vi "Monitor_Temp.vi"(2 "Debug Mode":bool, 3 "Elapsed Time (s)":dbl, 4 "State":enum16{"Edit", "Start", "Run", "End", "Idle"}(ring), 5 "Argument List In":string[](array[string])) -> (0 "Status Out":string, 1 "Argument List Out":string[](array[string]))   [LabVIEW 2011]
panel:
  in  "Cancel":bool
  in  "OK":bool
  out "Temperature":dbl
  out "Read Cycle":dbl
  out "Timer":dbl
  out "Previous Time":dbl
  in  "Target (C)":dbl
  # "Wait for this target \nto be reached."
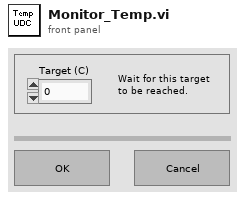
[diagram p1: front panel]
types:
  T1 = enum16{"Discrete", "Continuous", "Instantaneous"}
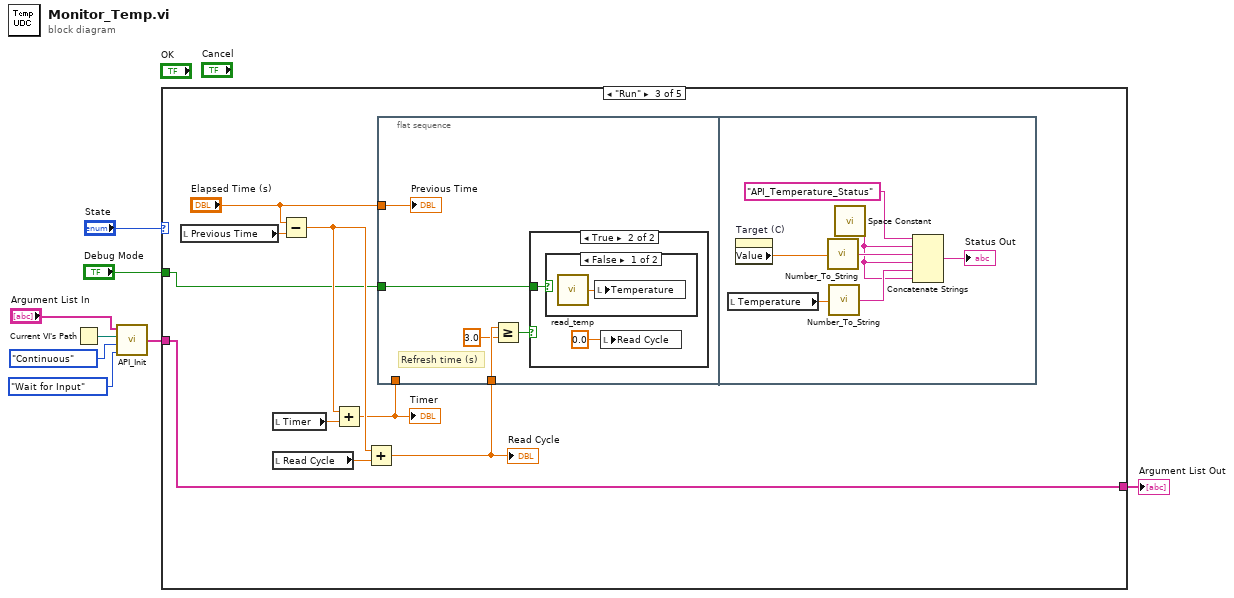
[diagram p0: block diagram]
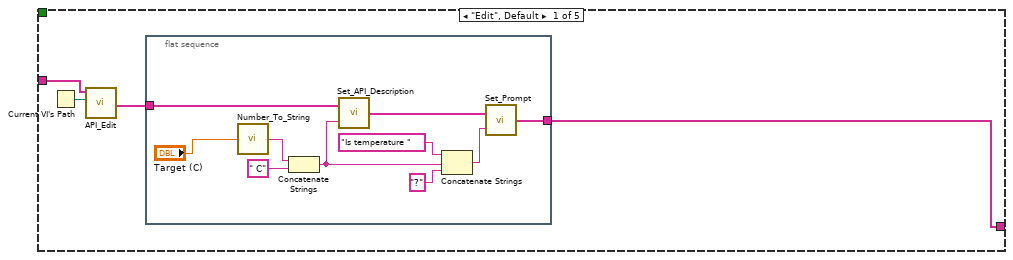
[diagram p2: hidden frame]
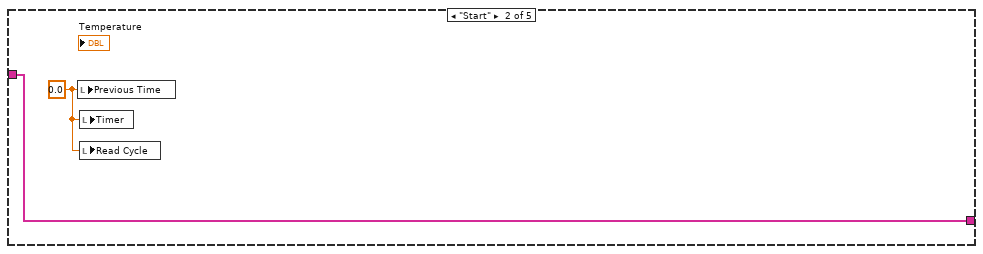
[diagram p3: hidden frame]
diagram:
  n1 = Current VI's Path() -> (path=w5:path)
  n2 = call "API_Init.vi"("API Option"=enum16{"None", "Blocking", "Wait for Input"}."Wait for Input", "API Mode"=T1."Continuous", "VI Path"=w5, "Argument List In"="Argument List In") -> ("Argument List Out"=w2:string[])
  n3 = case shown="\"Run\"" "State" {
    tunnel: [w9 w24 w33 w49 w50] -> w7
    tunnel: w2 -> [w11 w24 w33 w49 w50]
    tunnel: "Debug Mode" -> [_ _ w25 _ _]
    frame "Edit", Default {
      n4 = Current VI's Path() -> (path=w12:path)
      n5 = call "API_Edit.vi"("VI Path"=w12, "Argument List In"=w11) -> ("Argument List Out"=w10:string[])  [unwired: 2 in]
      n6 = flat-sequence {
        tunnel: w10 -> [w16]
        tunnel: [w14] -> w9
        frame #0 {
          n7 = call "Number_To_String.vi"("Number"="Target (C)") -> ("String"=w15:string)
          n8 = Concatenate Strings(w15, " C" ("string")) -> (w20:string)
          n9 = call "Set_API_Description.vi"("Description"=w20, "Argument List In"=w16) -> ("Argument List Out"=w21:string[])
          n10 = Concatenate Strings("Is temperature " ("Prompt"), w20, "?" ("string")) -> (w17:string)
          n11 = call "Set_Prompt.vi"("Prompt"=w17, "Argument List In"=w21) -> ("Argument List Out"=w14:string[])
        }
      }
    }
    frame "Start" {
      w23 = 0.0 ("Previous Time")
      n12 = local write "Previous Time"(w23) -> ()
      n13 = local write "Timer"(w23) -> ()
      n14 = local write "Read Cycle"(w23) -> ()
    }
    frame "Run" {
      n15 = local read "Previous Time"() -> (w31:dbl)
      n16 = local read "Timer"() -> (w30:dbl)
      n17 = local read "Read Cycle"() -> (w29:dbl)
      n18 = Subtract(x="Elapsed Time (s)", y=w31) -> (x-y=w28:dbl)
      n19 = Add(x=w28, y=w30) -> (x+y=w26:dbl)
      "Timer" <- w26
      n20 = Add(x=w28, y=w29) -> (x+y=w27:dbl)
      "Read Cycle" <- w27
      n21 = flat-sequence {
        tunnel: w26 -> [_]
        tunnel: w27 -> [w37]
        tunnel: "Elapsed Time (s)" -> [w38]
        tunnel: w25 -> [w34]
        frame #0 {
          # "Refresh time (s)"
          n22 = Greater Or Equal?(x=w37, y=3.0) -> (x >= y?=w35:bool)
          n23 = case shown="True" w35 {
            tunnel: w34 -> [_ w39]
            frame False {
            }
            frame True {
              n24 = case shown="False" w39 {
                frame False {
                  n25 = call "read_temp.vi"() -> ("Temperature (C)"=w41:dbl)  [unwired: 1 out]
                  n26 = local write "Temperature"(w41) -> ()
                }
                frame True {
                }
              }
              n27 = local write "Read Cycle"(0.0 ("Read Cycle")) -> ()
            }
          }
          "Previous Time" <- w38
        }
        frame #1 {
          n28 = local read "Temperature"() -> (w42:dbl)
          n29 = property on="Target (C)" class="DigNum (strict)"() -> ("Value"=w44:dbl)  [unwired: 2 in, 2 out]
          n30 = call "Number_To_String.vi"("Number"=w44) -> ("String"=w48:string)
          n31 = call "Number_To_String.vi"("Number"=w42) -> ("String"=w47:string)
          n32 = call <vilib>:"Space Constant.vi"() -> ("String"=w45:string)
          n33 = Concatenate Strings("API_Temperature_Status" ("string"), w45, w48, w45, w47, w45) -> (→"Status Out":string)
        }
      }
    }
    frame "End" {
    }
    frame "Idle" {
    }
  }
  "Argument List Out" <- w7
